vi "Read Single Waveform with trigger.vi"(6 "VISA Trigger":refnum<visa-resource-name>, 8 "error in (no error)":errorcluster, 9 "Maximum Time (10000 ms)":u32=10000, 10 "Channel (0: Channel 1)":u16(ring) format="%#_5f" items=["Channel 1", "Channel 2", "Channel 3", "Channel 4", "Math 1", "Math 2", "Math 3", "Math 4", "Reference 1", "Reference 2", "Reference 3", "Reference 4"], 11 "VISA OSC":refnum<visa-resource-name>) -> (0 "error out":errorcluster, 2 "Waveform Data":waveform(dbl)(graph)={"t0"=timestamp(1.815305999999491e-07 s since 1904-01-01), "dt"=5e-07, "Y"=array[10000 elements]}, 3 "VISA resource name out":refnum<visa-resource-name>)   [LabVIEW 2011, in "Tektronix 7000 Series.lvlib"]
doc: "Initiates an acquisition on all channels that you enabled with the Configure Channel VI. This VI waits for the acquisition to complete and returns the waveform for the <B>Channel</B> you specify. If the oscilloscope does not complete the acquisition within the <B>Maximum Time</B> period, this VI returns a timeout error. A timeout error often occurs because the acquisition is not triggered. For example, if the trigger level is out of range of the waveform, the acquisition is not triggered.\n\nRun the Fetch Waveform VI to obtain the waveforms for each of the remaining enabled <B>Channels</B> without initiating another acquisition.\n\n<B>Note:</B> If the instrument does not support autocompensation for probe attenuation, you might need to adjust the scaling of the <B>Waveform Data</B> accordingly. You can adjust the scaling using the Configure Channel VI or manually multiplying the <B>Waveform Data</B> by the probe attenuation."
uses:
  <instrlib>/Tektronix 7000 Series/Tektronix 7000 Series.lvlib
  <instrlib>/Tektronix 7000 Series/Public/Data/Low Level/Fetch (Waveform).vi
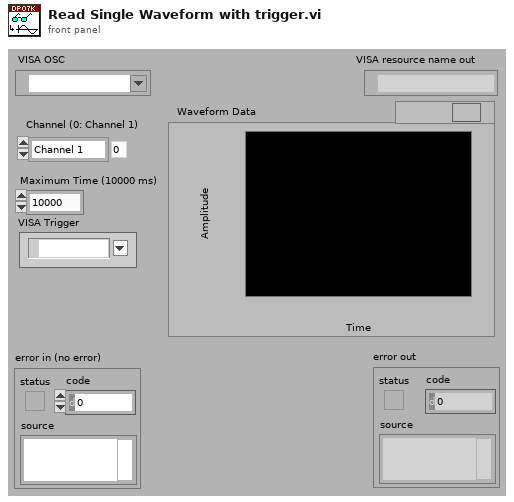
[diagram p1: front panel]
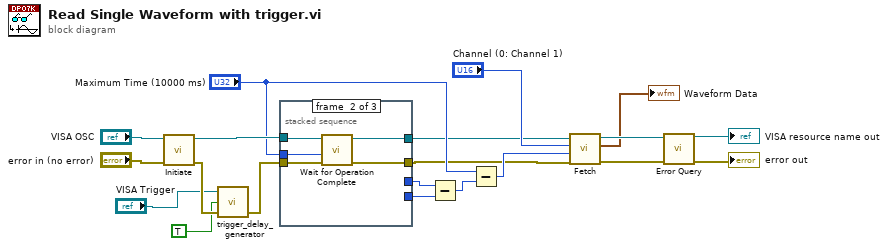
[diagram p0: block diagram]
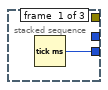
[diagram p2: hidden frame]
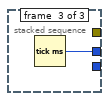
[diagram p3: hidden frame]
diagram:
  n1 = call <instrlib>:"Initiate.vi"("error in (no error)"="error in (no error)", "VISA resource name"="VISA OSC") -> ("error out"=w4:errorcluster, "VISA resource name out"=w12:refnum<visa-resource-name>)  [unwired: 8 in]
  n2 = call "trigger_delay_generator.vi"("error in (no error)"=w4, "Boolean"=TRUE, "VISA resource name"="VISA Trigger") -> ("error out"=w3:errorcluster)  [unwired: 1 in, 1 out]
  n3 = stacked-sequence {
    tunnel: w12 -> [_ w26 _]
    tunnel: w3 -> [_ w25 _]
    tunnel: [_ _ w27] -> w11
    tunnel: [w21 _ _] -> w10
    tunnel: "Maximum Time (10000 ms)" -> [_ w24 _]
    tunnel: [_ w23 _] -> w6
    tunnel: [_ w22 _] -> w5
    frame #0 {
      n4 = Tick Count (ms)() -> (millisecond timer value=w21:u32)
    }
    frame #1 {
      n5 = call <instrlib>:"Wait for Operation Complete.vi"("error in (no error)"=w25, "Maximum Time (2000ms)"=w24, "VISA resource name"=w26) -> ("error out"=w22:errorcluster, "VISA resource name out"=w23:refnum<visa-resource-name>)  [unwired: 7 in]
    }
    frame #2 {
      n6 = Tick Count (ms)() -> (millisecond timer value=w27:u32)
    }
  }
  n7 = Subtract(x=w11, y=w10) -> (x-y=w9:u32)
  n8 = Subtract(x="Maximum Time (10000 ms)", y=w9) -> (x-y=w7:u32)
  n9 = call-poly <instrlib>:"Fetch.vi"("error in (no error)"=w5, "Maximum Time (10000ms)"=w7, "Channel (0:Channel1)"="Channel (0: Channel 1)", "VISA resource name"=w6) -> ("error out"=w17:errorcluster, "Waveform Data"=→"Waveform Data":waveform(dbl), "VISA resource name out"=w18:refnum<visa-resource-name>)  [unwired: 5 in]
  n10 = call <instrlib>:"Error Query.vi"("error in (no error)"=w17, "VISA resource name"=w18) -> ("error out"=→"error out":errorcluster, "VISA resource name out"=→"VISA resource name out":refnum<visa-resource-name>)  [unwired: 6 in, 2 out]
